vi "CameraGetData.vi"(8 "error in (no error)":errorcluster, 10 "keep open?":bool, 11 "CameraBase in":refnum<class "CameraBase.lvclass">) -> (0 "error out":errorcluster, 2 "image_data":u16[][][](array[numeric]), 3 "CameraBase out":refnum<class "CameraBase.lvclass">)   [LabVIEW 2010, in "CameraBase.lvclass"]
uses:
  CameraBase.lvclass
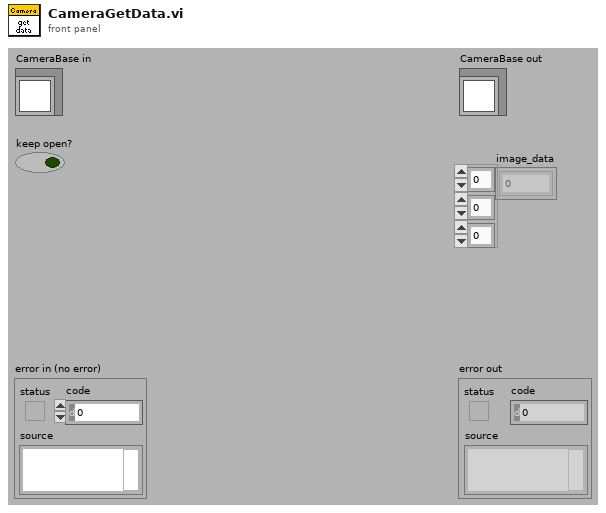
[diagram p1: front panel]
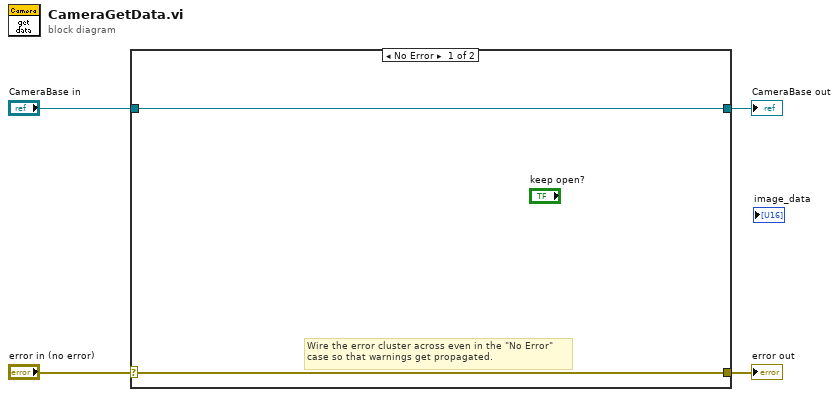
[diagram p0: block diagram]
diagram:
  n1 = case shown="No Error" "error in (no error)" {
    selector: "error in (no error)" -> [w5 w8]
    tunnel: [w5 w8] -> w3
    tunnel: [w6 w7] -> w1
    tunnel: "CameraBase in" -> [w6 w7]
    frame No Error {
      # "Wire the error cluster across even in the \"No Error\"\ncase so that warnings get propagated."
    }
    frame Error {
    }
  }
  "error out" <- w3
  "CameraBase out" <- w1
